vi "PH_PLH-AccessInformation.ProcCases.vi"(0 "i ref in":refnum<vi>, 1 "selector":string, 2 "Data":T1, 3 "call cluster":T2={"Object"="", "Selector"="", "CallType"=enum."synchronous", "Async Object"="", "Async Selector"="", "Data Descriptor"="", "Data"=[], "Error #"=0, "Expire"=0}, 5 "error in (no error)":errorcluster) -> (14 "i ref out":refnum<vi>, 17 "answer cluster":T2={"Object"="", "Selector"="", "CallType"=enum."synchronous", "Async Object"="", "Async Selector"="", "Data Descriptor"="", "Data"=[], "Error #"=0, "Expire"=0}, 19 "error out":errorcluster)   [LabVIEW 2014, in "PH_PLH-AccessInformation.lvlib"]
doc: "This method is called by a process from within the default case in the event loop. The methods of a class that are linked to events will be called from THIS method. Add your code here."
uses:
  PH_PLH-AccessInformation.lvlib
  CSCore/CSSystem/CoreDefs/CoreDefs.call_type.ctl
  CSCore/BaseProcess/BaseProcess.descriptor string definition.ctl
  CSCore/CSSystem/CoreDefs/CoreDefs.rawDataType.ctl
  CSCore/CSSystem/CoreLib/CoreLib.string 2 byte array.vi
  CSCore/BaseProcess/BaseProcess.lvlib
  PH_Common/PH_Common.lvlib
  CSCore/CAEObj/CAEObj.lvlib
  CSCore/CSSystem/CoreLib/CoreLib.lvlib
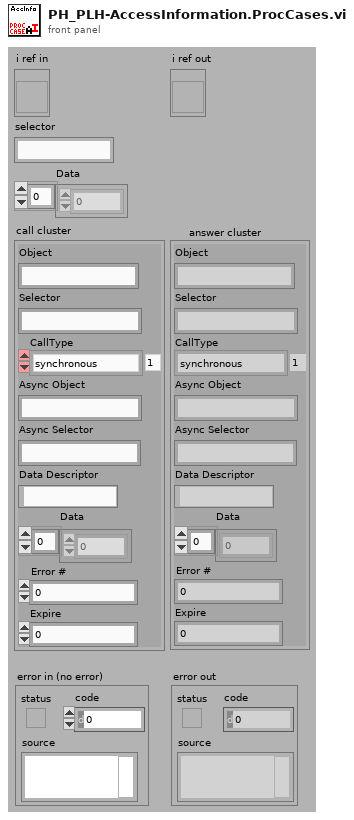
[diagram p1: front panel]
types:
  T1 = typedef "CoreDefs.rawDataType.ctl" = i8[]
  T2 = typedef "CoreDefs.call_type.ctl" = cluster{"Object":string, "Selector":string, "CallType":enum16{"simple", "synchronous", "asynchronous"}, "Async Object":string, "Async Selector":string, "Data Descriptor":T3, "Data":T1, "Error #":i32, "Expire":u32}
  T3 = typedef "BaseProcess.lvlib/BaseProcess.descriptor string definition.ctl" = string
  T4 = typedef "PH_PLH-AccessInformation.lvlib/PH_PLH-AccessInformation.i attribute.ctl" = cluster{"GUI Refs":cluster{"Ref Shotmode":refnum<vi>, "Ref Searchmode":refnum<vi>}, "Shotmode":i32, "Searchmode":i32}
  T5 = enum16{"no info", "free access", "Searchmode", "Shotmode"}
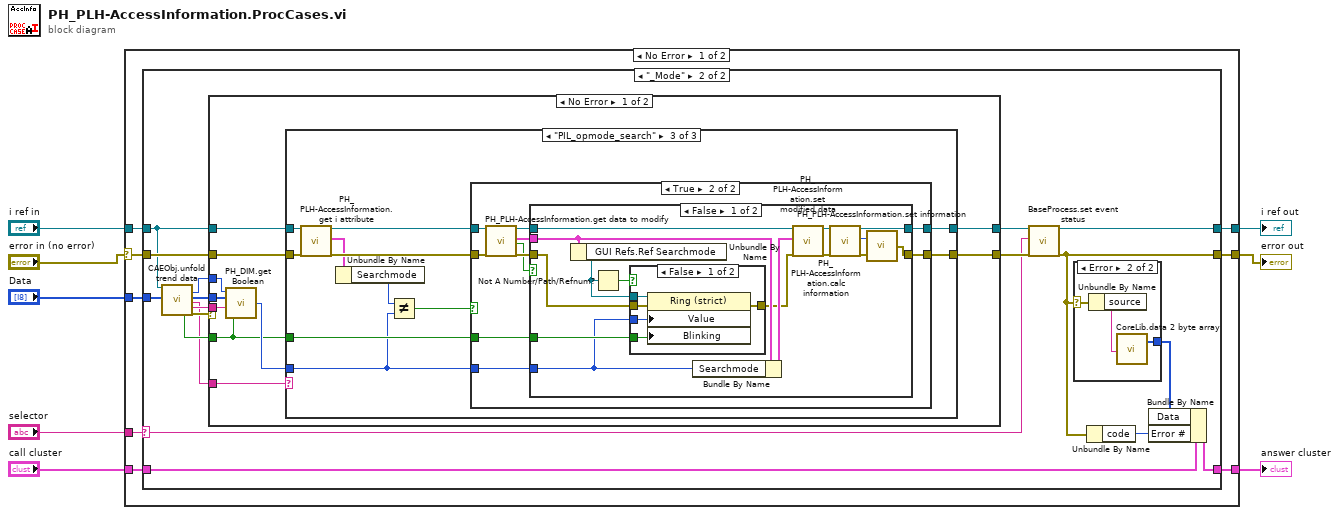
[diagram p0: block diagram]
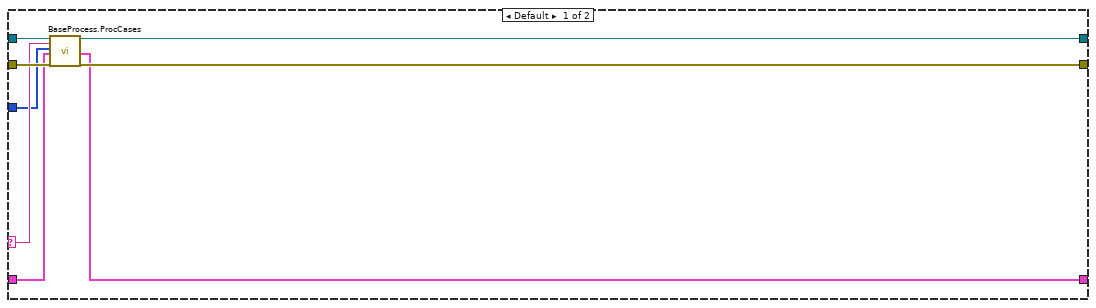
[diagram p2: hidden frame]
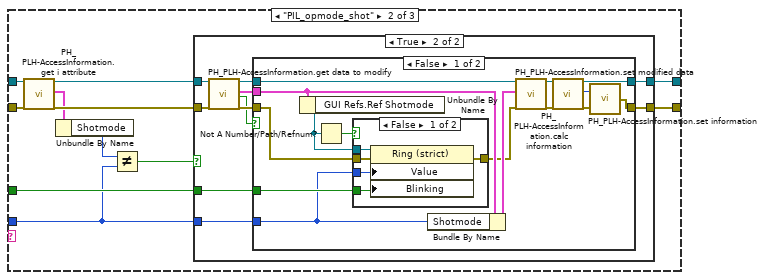
[diagram p5: hidden frame]
diagram:
  n1 = case shown="No Error" "error in (no error)" {
    selector: "error in (no error)" -> [w9 w153]
    tunnel: "selector" -> [w16 _]
    tunnel: [w15 w152] -> w7
    tunnel: "call cluster" -> [w14 w152]
    tunnel: "i ref in" -> [w13 w154]
    tunnel: [w12 w154] -> w4
    tunnel: [w11 w153] -> w3
    tunnel: "Data" -> [w10 _]
    frame No Error {
      n2 = case shown="\"_Mode\"" w16 {
        selector: w16 -> [w19 w28]
        tunnel: w13 -> [w18 w40]
        tunnel: [w24 w29] -> w12
        tunnel: w14 -> [w20 w27]
        tunnel: [w21 w26] -> w15
        tunnel: w9 -> [w23 w42]
        tunnel: [w22 w30] -> w11
        tunnel: w10 -> [w17 w41]
        frame Default {
          n3 = call "BaseProcess.ProcCases.vi"("i ref in"=w18, "selector"=w19, "Data"=w17, "call cluster"=w20, "error in (no error)"=w23) -> ("i ref out"=w24:refnum<vi>, "answer cluster"=w21:T2, "error out"=w22:errorcluster)  [unwired: 12 in]
        }
        frame "_Mode" {
          n4 = call "CAEObj.unfold trend data.vi"("i ref in"=w40, "raw trend data"=w41) -> ("quality"=w38:i32, "no link"=w37:bool, "data"=w36:i8[], "serviceName"=w25:string, "typeDescriptor"=w35:string, "error out"=w39:errorcluster)  [unwired: 9 in, 3 out]
          n5 = case shown="No Error" w39 {
            tunnel: [w48 w151] -> w32
            tunnel: w40 -> [w52 w151]
            tunnel: w42 -> [w51 w150]
            tunnel: [w47 w150] -> w31
            tunnel: w38 -> [w55 _]
            tunnel: w37 -> [w49 _]
            tunnel: w36 -> [w54 _]
            tunnel: w35 -> [w53 _]
            tunnel: w25 -> [w46 _]
            frame No Error {
              n6 = call "PH_DIM.get Boolean.vi"("no link"=w49, "typeDescriptor"=w53, "data"=w54, "quality"=w55) -> ("Value"=w50:i32)
              n7 = case shown="\"PIL_opmode_search\"" w46 {
                tunnel: w52 -> [w57 w63 w109]
                tunnel: w51 -> [w56 w68 w114]
                tunnel: w50 -> [_ w59 w105]
                tunnel: w49 -> [_ w67 w113]
                tunnel: [w57 w66 w112] -> w48
                tunnel: [w56 w65 w111] -> w47
                frame Default {
                }
                frame "PIL_opmode_shot" {
                  n8 = call "PH_PLH-AccessInformation.get i attribute.vi"("i ref in"=w63, "error in (no error)"=w68) -> ("i ref out"=w62:refnum<vi>, "i attribute"=w61:T4, "error out"=w64:errorcluster)  [unwired: 15 in]
                  n9 = Unbundle By Name(w61) -> ("Shotmode"=w60:i32)
                  n10 = Not Equal?(x=w60, y=w59) -> (x != y?=w58:bool)
                  n11 = case shown="True" w58 {
                    tunnel: w67 -> [_ w76]
                    tunnel: [w70 w75] -> w66
                    tunnel: [w69 w74] -> w65
                    tunnel: w64 -> [w69 w73]
                    tunnel: w62 -> [w70 w72]
                    tunnel: w59 -> [_ w71]
                    frame False {
                    }
                    frame True {
                      n12 = call "PH_PLH-AccessInformation.get data to modify.vi"("i ref in"=w72, "error in (no error)"=w73) -> ("i ref out"=w79:refnum<vi>, "i attribute"=w77:T4, "timed out"=w78:bool, "error out"=w80:errorcluster)  [unwired: 14 in]
                      n13 = case shown="False" w78 {
                        tunnel: w80 -> [w93 w102]
                        tunnel: w79 -> [w90 w103]
                        tunnel: [w83 w103] -> w75
                        tunnel: [w88 w102] -> w74
                        tunnel: w77 -> [w94 _]
                        tunnel: w71 -> [w91 _]
                        tunnel: w76 -> [w92 _]
                        frame False {
                          n14 = Unbundle By Name(w94) -> ("GUI Refs.Ref Shotmode"=w82:refnum<vi>)
                          n15 = Not A Number/Path/Refnum?(number/path/refnum=w82) -> (NaN/Path/Refnum?=w81:bool)
                          n16 = case shown="False" w81 {
                            tunnel: w93 -> [w100 w101]
                            tunnel: [w99 w101] -> w89
                            tunnel: w82 -> [w98 _]
                            tunnel: w91 -> [w97 _]
                            tunnel: w92 -> [w96 _]
                            frame False {
                              n17 = property class="Ring (strict)"(reference=w98, error in=w100, "Value"=w97, "Blinking"=w96) -> (error out=w99:errorcluster)  [unwired: 1 out]
                            }
                            frame True {
                            }
                          }
                          n18 = Bundle By Name(cluster=w94, "Shotmode"=w91) -> (w95:T4)
                          n19 = call "PH_PLH-AccessInformation.set modified data.vi"("i ref in"=w90, "i attribute"=w95, "error in (no error)"=w89) -> ("i ref out"=w87:refnum<vi>, "error out"=w86:errorcluster)  [unwired: 15 in]
                          n20 = call "PH_PLH-AccessInformation.calc information.vi"("i ref in"=w87, "error in"=w86) -> ("i ref out"=w83:refnum<vi>, "Mode"=w84:T5, "error out"=w85:errorcluster)  [unwired: 15 in]
                          n21 = call "PH_PLH-AccessInformation.set information.vi"("error in(no error)"=w85, "Mode"=w84) -> ("error out"=w88:errorcluster)
                        }
                        frame True {
                        }
                      }
                    }
                  }
                }
                frame "PIL_opmode_search" {
                  n22 = call "PH_PLH-AccessInformation.get i attribute.vi"("i ref in"=w109, "error in (no error)"=w114) -> ("i ref out"=w108:refnum<vi>, "i attribute"=w107:T4, "error out"=w110:errorcluster)  [unwired: 15 in]
                  n23 = Unbundle By Name(w107) -> ("Searchmode"=w106:i32)
                  n24 = Not Equal?(x=w106, y=w105) -> (x != y?=w104:bool)
                  n25 = case shown="True" w104 {
                    tunnel: w113 -> [_ w122]
                    tunnel: [w116 w121] -> w112
                    tunnel: [w115 w120] -> w111
                    tunnel: w110 -> [w115 w119]
                    tunnel: w108 -> [w116 w118]
                    tunnel: w105 -> [_ w117]
                    frame False {
                    }
                    frame True {
                      n26 = call "PH_PLH-AccessInformation.get data to modify.vi"("i ref in"=w118, "error in (no error)"=w119) -> ("i ref out"=w125:refnum<vi>, "i attribute"=w123:T4, "timed out"=w124:bool, "error out"=w126:errorcluster)  [unwired: 14 in]
                      n27 = case shown="False" w124 {
                        tunnel: w126 -> [w139 w148]
                        tunnel: w125 -> [w136 w149]
                        tunnel: [w129 w149] -> w121
                        tunnel: [w134 w148] -> w120
                        tunnel: w123 -> [w140 _]
                        tunnel: w117 -> [w137 _]
                        tunnel: w122 -> [w138 _]
                        frame False {
                          n28 = Unbundle By Name(w140) -> ("GUI Refs.Ref Searchmode"=w128:refnum<vi>)
                          n29 = Not A Number/Path/Refnum?(number/path/refnum=w128) -> (NaN/Path/Refnum?=w127:bool)
                          n30 = case shown="False" w127 {
                            tunnel: w139 -> [w146 w147]
                            tunnel: [w145 w147] -> w135
                            tunnel: w128 -> [w144 _]
                            tunnel: w137 -> [w143 _]
                            tunnel: w138 -> [w142 _]
                            frame False {
                              n31 = property class="Ring (strict)"(reference=w144, error in=w146, "Value"=w143, "Blinking"=w142) -> (error out=w145:errorcluster)  [unwired: 1 out]
                            }
                            frame True {
                            }
                          }
                          n32 = Bundle By Name(cluster=w140, "Searchmode"=w137) -> (w141:T4)
                          n33 = call "PH_PLH-AccessInformation.set modified data.vi"("i ref in"=w136, "i attribute"=w141, "error in (no error)"=w135) -> ("i ref out"=w133:refnum<vi>, "error out"=w132:errorcluster)  [unwired: 15 in]
                          n34 = call "PH_PLH-AccessInformation.calc information.vi"("i ref in"=w133, "error in"=w132) -> ("i ref out"=w129:refnum<vi>, "Mode"=w130:T5, "error out"=w131:errorcluster)  [unwired: 15 in]
                          n35 = call "PH_PLH-AccessInformation.set information.vi"("error in(no error)"=w131, "Mode"=w130) -> ("error out"=w134:errorcluster)
                        }
                        frame True {
                        }
                      }
                    }
                  }
                }
              }
            }
            frame Error {
            }
          }
          n36 = call "BaseProcess.set event status.vi"("i ref in"=w32, "EventStatus"=w28, "error in (no error)"=w31) -> ("i ref out"=w29:refnum<vi>, "error out"=w30:errorcluster)  [unwired: 14 in, 1 out]
          n37 = case shown="Error" w30 {
            selector: w30 -> [_ w45]
            tunnel: [_ w43] -> w33
            frame No Error {
            }
            frame Error {
              n38 = Unbundle By Name(w45) -> ("source"=w44:string)
              n39 = call-poly "CoreLib.data 2 byte array.vi"("string"=w44) -> ("byteArray out"=w43:T1)  [unwired: 18 in]
            }
          }
          n40 = Unbundle By Name(w30) -> ("code"=w34:i32)
          n41 = Bundle By Name(cluster=w27, "Data"=w33, "Error #"=w34) -> (w26:T2)
        }
      }
    }
    frame Error {
    }
  }
  "answer cluster" <- w7
  "i ref out" <- w4
  "error out" <- w3
